vi "F Dwf Digital Spi Write Read16.vi"(0 "hdwf":i32, 1 "cTX":i32, 2 "cRX":i32, 5 "cDQ":i32, 7 "cBitPerWord":i32, 9 "rgTX":u16, 11 "error in (no error)":errorcluster, 12 "rgRX":u16) -> (4 "function return":i32, 10 "rgTX out":u16, 14 "rgRX out":u16, 15 "error out":errorcluster)   [LabVIEW 2021, in "Olasdwf.lvlib"]
doc: "DWFAPI int FDwfDigitalSpiWriteRead16(HDWF hdwf, int cDQ, int cBitPerWord, unsigned short *rgTX, int cTX, unsigned short *rgRX, int cRX);"
uses:
  Olasdwf.lvlib
  Windows/System32/dwf.dll
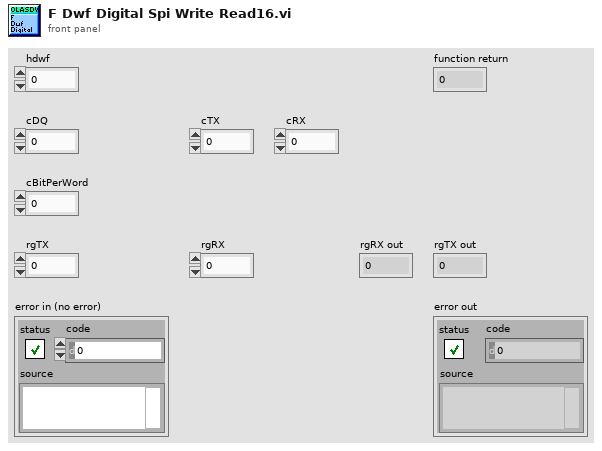
[diagram p1: front panel]
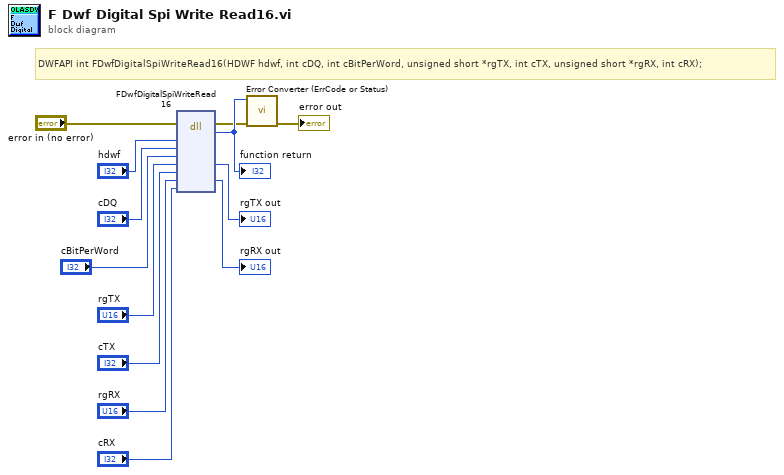
[diagram p0: block diagram]
diagram:
  # "DWFAPI int FDwfDigitalSpiWriteRead16(HDWF hdwf, int cDQ, int cBitPerWord, unsigned short *rgTX, int cTX, unsigned short *rgRX, int cRX);"
  n1 = dll-call lib="/Windows/System32/dwf.*" fn="FDwfDigitalSpiWriteRead16"(error in="error in (no error)", "hdwf"="hdwf", "cDQ"="cDQ", "cBitPerWord"="cBitPerWord", "rgTX"="rgTX", "cTX"="cTX", "rgRX"="rgRX", "cRX"="cRX") -> (error out=w2:errorcluster, w13:i32, "rgTX"=→"rgTX out":u16, "rgRX"=→"rgRX out":u16)  [unwired: 7 in, 1 out]
  "function return" <- w13
  n2 = call "Error Converter (ErrCode or Status).vi"("error in (no error)"=w2, "error code"=w13) -> ("error out"=→"error out":errorcluster)  [unwired: 9 in]
